vi "Get QM param from PGserver.vi"(6 "conninfo":T1={"host"="localhost", "port"="5432", "client_encoding"="WIN1251", "dbname"="data", "user"="postgres", "password"=""}, 8 "error in (no error)":errorcluster, 9 "ParamColumns":string[](array[string])=["value", "value_range_min", "value_range_max", "d", "fname", "value_units", "fcode_unpack", "fcodef"], 10 "ParamTable":string="par_3", 11 "Parameters":string[](array[string])) -> (0 "error out":errorcluster, 2 "Names table":string[][](array[string]), 3 "Parameters table":dbl[][](array[numeric]))   [LabVIEW 2019, in "Valves.lvlib"]
uses:
  Valves.lvlib
  Database/ctl/Coninfo.ctl
  Database/PostgreSQL2LabVIEW/libpqlv/src/PQfinish.vi
  Database/PostgreSQL2LabVIEW/libpqlv/src/PQconnectdb.vi
  Database/PostgreSQL2LabVIEW/libpqlv/src/PQerrorMessage.vi
  Database/PostgreSQL2LabVIEW/libpqlv/src/PQstatus.vi
  <vilib>/dlg_ctls.llb/Space Constant.vi
  Database/Progress.vi
  Database/PostgreSQL.lvlib
  Database/PostgreSQL2LabVIEW/libpqUtility/libpqutility.lvlib
  Database/PostgreSQL2LabVIEW/libpqUtility64/libpqutility64.lvlib
panel:
  out "PQStatus":T2(ring)
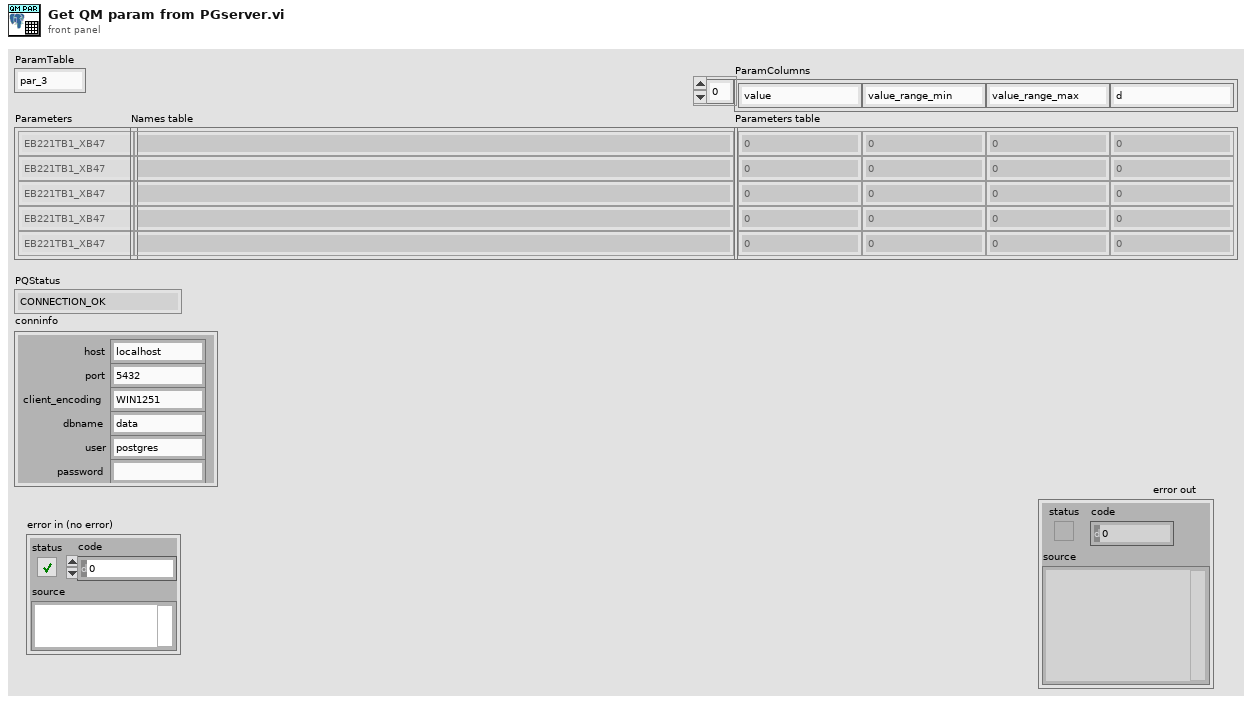
[diagram p1: front panel]
types:
  T1 = typedef "PostgreSQL.lvlib/Coninfo.ctl" = cluster{"host":string, "port":string, "client_encoding":string, "dbname":string, "user":string, "password":string}
  T2 = enum32{"CONNECTION_OK", "CONNECTION_BAD", "CONNECTION_STARTED", "CONNECTION_MADE", "CONNECTION_AWAITING_RESPONSE", "CONNECTION_AUTH_OK", "CONNECTION_SETENV", "CONNECTION_SSL_STARTUP", "CONNECTION_NEEDED"}
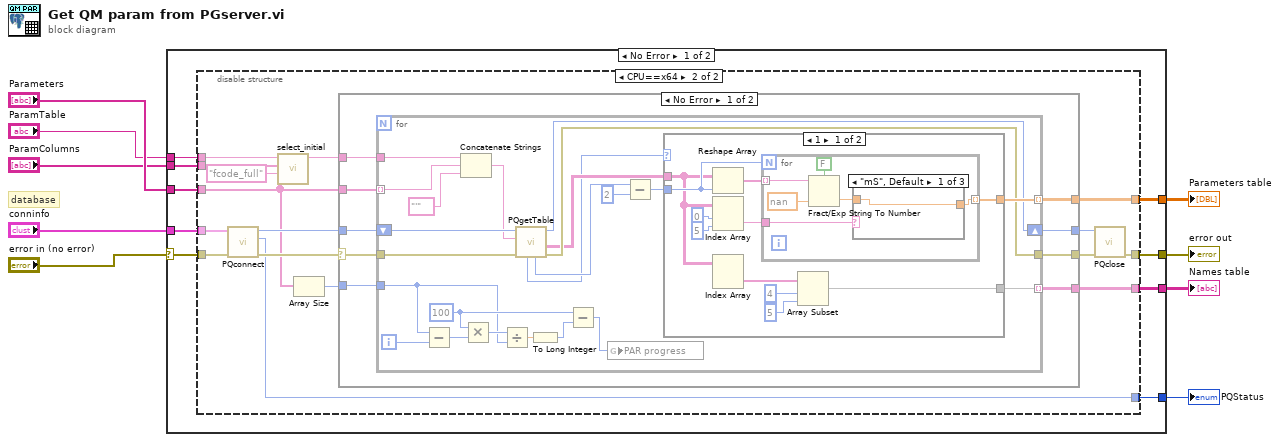
[diagram p0: block diagram]
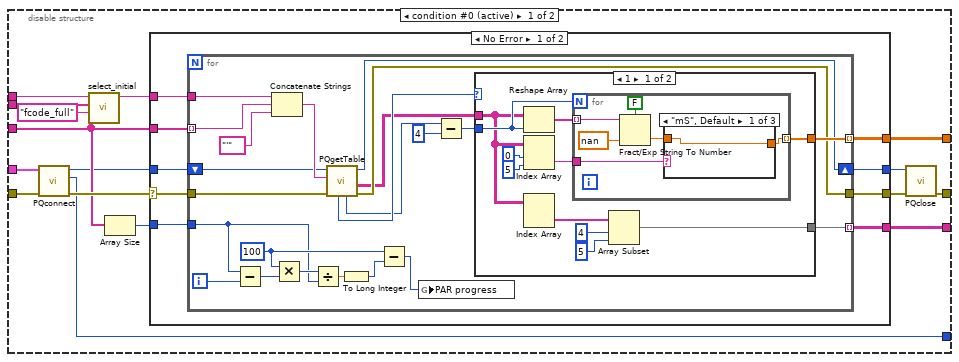
[diagram p2: hidden frame]
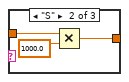
[diagram p3: hidden frame]
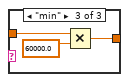
[diagram p4: hidden frame]
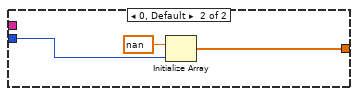
[diagram p5: hidden frame]
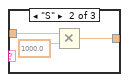
[diagram p7: hidden frame]
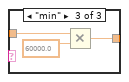
[diagram p8: hidden frame]
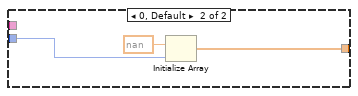
[diagram p9: hidden frame]
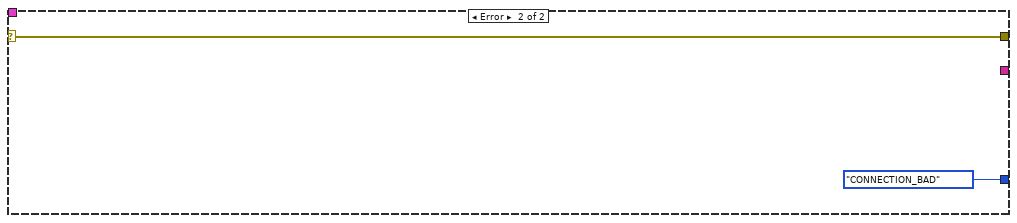
[diagram p11: hidden frame]
diagram:
  # "database"
  n1 = case shown="No Error" "error in (no error)" {
    selector: "error in (no error)" -> [w11 w174]
    tunnel: "Parameters" -> [w18 _]
    tunnel: "ParamTable" -> [w16 _]
    tunnel: "ParamColumns" -> [w15 _]
    tunnel: [w17 _] -> w6
    tunnel: [w14 w174] -> w5
    tunnel: [w13 _] -> w4
    tunnel: "conninfo" -> [w12 _]
    tunnel: [w10 T2."CONNECTION_BAD" ("PQStatus")] -> w1
    frame No Error {
      n2 = disable-structure shown="CPU==x64" {
        disable-tunnel: w18 -> [w33 w102]
        disable-tunnel: [w32 w96] -> w17
        disable-tunnel: w16 -> [w30 w104]
        disable-tunnel: w15 -> [w29 w103]
        disable-tunnel: [w28 w97] -> w14
        disable-tunnel: [w27 w98] -> w13
        disable-tunnel: w12 -> [w26 w101]
        disable-tunnel: w11 -> [w25 w100]
        disable-tunnel: [w19 w99] -> w10
        frame condition #0 (active) {
          n3 = call "PQconnect.vi"("error in (no error)"=w25, "conninfo"=w26) -> ("error out"=w34:errorcluster, "PQStatus"=w19:T2, "conn"=w21:u32)  [unwired: 7 in]
          n4 = call "select_initial.vi"("Column name"="fcode_full", "Column table"=w29, "table"=w30) -> ("parameters"=w23:string)  [unwired: 7 in, 1 out]
          n5 = Array Size(array=w33) -> (size(s)=w24:i32)
          n6 = case shown="No Error" w34 {
            selector: w34 -> [w42 w95]
            tunnel: w33 -> [w41 _]
            tunnel: [w39 _] -> w32
            tunnel: [w36 _] -> w27
            tunnel: w24 -> [w35 _]
            tunnel: w21 -> [w43 w94]
            tunnel: w23 -> [w40 _]
            tunnel: [w37 w95] -> w31
            tunnel: [w38 w94] -> w20
            frame No Error {
              n7 = for {
                tunnel: [w54] -> w39 mode=indexing
                tunnel: w42 -> [w47]
                tunnel: w35 -> [w56]
                tunnel: w41 -> [w65] mode=indexing
                tunnel: w40 -> [w66]
                tunnel: [w53] -> w36 mode=indexing
                tunnel: [w46] -> w37
                shift-right: [w44] -> w38
                shift-left: w43 -> [w50]
                i -> [w57]
                w61 = 100 ("y")
                n8 = Subtract(x=w56, y=w57) -> (x-y=w60:i32)
                n9 = Concatenate Strings(w66, w65, "'" ("table")) -> (w51:string)
                n10 = Multiply(x=w61, y=w60) -> (x*y=w63:i32)
                n11 = Divide(x=w63, y=w56) -> (x/y=w59:dbl)
                n12 = call "PQgetTable.vi"("error in"=w47, "query"=w51, "conn"=w50) -> ("error out"=w46:errorcluster, "Data"=w45:string[][], "conn_out"=w44:u32, "PQnFields"=w48:i32, "PQnTuples"=w49:i32)  [unwired: 4 in]
                n13 = To Long Integer(number=w59) -> (32bit integer=w58:i32)
                n14 = Subtract(x=w61, y=w58) -> (x-y=w62:i32)
                n15 = global write "Progress.vi" "PAR progress"(w62) -> ()
                n16 = Subtract(x=w48, y=4) -> (x-y=w55:i32)
                n17 = case shown="1" w49 {
                  tunnel: [w77 w92] -> w54
                  tunnel: w55 -> [w75 w91]
                  tunnel: w45 -> [w68 _]
                  tunnel: [w74 _] -> w53
                  frame 1 {
                    n18 = Reshape Array(w68, w75) -> (w76:string[])
                    n19 = Index Array(array=w68, index (row)=0, index (col)=5) -> (element=w67:string)
                    n20 = Index Array(array=w68) -> (element=w71:string[])  [unwired: 2 in]
                    n21 = for {
                      N: w75 -> [_]
                      tunnel: w76 -> [w82] mode=indexing
                      tunnel: [w78] -> w77 mode=indexing
                      tunnel: w67 -> [w79]
                      n22 = Fract/Exp String To Number(use system decimal point (T)=FALSE, string=w82, default (0 dbl)=nan) -> (number=w80:dbl)  [unwired: 1 in, 1 out]
                      n23 = case shown="\"mS\", Default" w79 {
                        tunnel: w80 -> [w84 w87 w90]
                        tunnel: [w84 w85 w88] -> w78
                        frame "mS", Default {
                        }
                        frame "S" {
                          n24 = Multiply(x=w87, y=1000.0) -> (x*y=w85:dbl)
                        }
                        frame "min" {
                          n25 = Multiply(x=w90, y=60000.0) -> (x*y=w88:dbl)
                        }
                      }
                    }
                    n26 = Array Subset(array=w71, index=4, length=5) -> (w74:string[])
                  }
                  frame 0, Default {
                    n27 = Initialize Array(nan, w91) -> (w92:dbl[])
                  }
                }
              }
            }
            frame Error {
            }
          }
          n28 = call "PQclose.vi"("error in (no error)"=w31, "conn"=w20) -> ("error out"=w28:errorcluster)  [unwired: 9 in]
        }
        frame condition #1 {
          n29 = call "PQconnect.vi"("error in (no error)"=w100, "conninfo"=w101) -> ("error out"=w111:errorcluster, "PQStatus"=w99:T2, "conn"=w106:u64)  [unwired: 7 in]
          n30 = call "select_initial.vi"("Column name"="fcode_full", "Column table"=w103, "table"=w104) -> ("parameters"=w108:string)  [unwired: 7 in, 1 out]
          n31 = Array Size(array=w102) -> (size(s)=w109:i32)
          n32 = case shown="No Error" w111 {
            selector: w111 -> [w119 w172]
            tunnel: w102 -> [w117 _]
            tunnel: [w120 _] -> w96
            tunnel: [w114 _] -> w98
            tunnel: w109 -> [w118 _]
            tunnel: w106 -> [w116 w171]
            tunnel: w108 -> [w115 _]
            tunnel: [w113 w172] -> w110
            tunnel: [w112 w171] -> w105
            frame No Error {
              n33 = for {
                tunnel: [w131] -> w120 mode=indexing
                tunnel: w119 -> [w126]
                tunnel: w118 -> [w133]
                tunnel: w117 -> [w142] mode=indexing
                tunnel: w115 -> [w143]
                tunnel: [w130] -> w114 mode=indexing
                tunnel: [w125] -> w113
                shift-right: [w121] -> w112
                shift-left: w116 -> [w128]
                i -> [w134]
                w138 = 100 ("y")
                n34 = Subtract(x=w133, y=w134) -> (x-y=w137:i32)
                n35 = Concatenate Strings(w143, w142, "'" ("table")) -> (w127:string)
                n36 = Multiply(x=w138, y=w137) -> (x*y=w140:i32)
                n37 = Divide(x=w140, y=w133) -> (x/y=w136:dbl)
                n38 = call "PQgetTable.vi"("error in"=w126, "query"=w127, "conn"=w128) -> ("error out"=w125:errorcluster, "Data"=w124:string[][], "conn_out"=w121:u64, "PQnFields"=w123:i64, "PQnTuples"=w122:i64)  [unwired: 4 in]
                n39 = To Long Integer(number=w136) -> (32bit integer=w135:i32)
                n40 = Subtract(x=w138, y=w135) -> (x-y=w139:i32)
                n41 = global write "Progress.vi" "PAR progress"(w139) -> ()
                n42 = Subtract(x=w123, y=2) -> (x-y=w132:i64)
                n43 = case shown="1" w122 {
                  tunnel: [w154 w169] -> w131
                  tunnel: w132 -> [w152 w168]
                  tunnel: w124 -> [w145 _]
                  tunnel: [w151 _] -> w130
                  frame 1 {
                    n44 = Reshape Array(w145, w152) -> (w153:string[])
                    n45 = Index Array(array=w145, index (row)=0, index (col)=5) -> (element=w144:string)
                    n46 = Index Array(array=w145) -> (element=w148:string[])  [unwired: 2 in]
                    n47 = for {
                      N: w152 -> [_]
                      tunnel: w153 -> [w159] mode=indexing
                      tunnel: [w155] -> w154 mode=indexing
                      tunnel: w144 -> [w156]
                      n48 = Fract/Exp String To Number(use system decimal point (T)=FALSE, string=w159, default (0 dbl)=nan) -> (number=w157:dbl)  [unwired: 1 in, 1 out]
                      n49 = case shown="\"mS\", Default" w156 {
                        tunnel: w157 -> [w161 w164 w167]
                        tunnel: [w161 w162 w165] -> w155
                        frame "mS", Default {
                        }
                        frame "S" {
                          n50 = Multiply(x=w164, y=1000.0) -> (x*y=w162:dbl)
                        }
                        frame "min" {
                          n51 = Multiply(x=w167, y=60000.0) -> (x*y=w165:dbl)
                        }
                      }
                    }
                    n52 = Array Subset(array=w148, index=4, length=5) -> (w151:string[])
                  }
                  frame 0, Default {
                    n53 = Initialize Array(nan, w168) -> (w169:dbl[])
                  }
                }
              }
            }
            frame Error {
            }
          }
          n54 = call "PQclose.vi"("error in (no error)"=w110, "conn"=w105) -> ("error out"=w97:errorcluster)  [unwired: 9 in]
        }
      }
    }
    frame Error {
    }
  }
  "error out" <- w5
  "Parameters table" <- w6
  "Names table" <- w4
  "PQStatus" <- w1
